vi "TypesetInsideMathmode.vi"(8 "Needs $$?":bool=TRUE, 11 "DirtyString":string) -> (0 "ChosenStringtype":string, 2 "Mathmode String":string, 3 "De-dollared String":string)   [LabVIEW 2014]
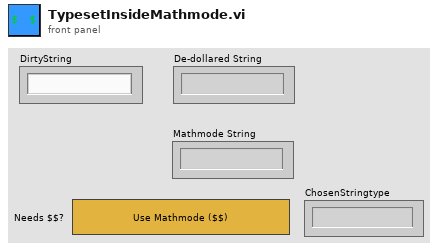
[diagram p1: front panel]
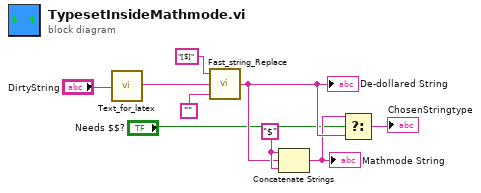
[diagram p0: block diagram]
diagram:
  w5 = "$" ("string")
  n1 = call "Text_for_latex.vi"("Input String"="DirtyString") -> ("Output String"=w6:string)
  n2 = call "Fast_string_Replace.vi"("Replace match with:"="", "Input String"=w6, "regular expression"="[$]") -> ("Output String"=w4:string)  [unwired: 2 out]
  "De-dollared String" <- w4
  n3 = Concatenate Strings(w5, w4, w5) -> (w3:string)
  "Mathmode String" <- w3
  n4 = Select(t=w3, s="Needs $$?", f=w4) -> (s? t:f=→"ChosenStringtype":string)
